vi "Mouse Monitor Terminate.vi"   [LabVIEW 2018]
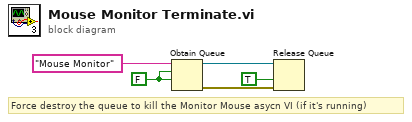
[diagram p0: block diagram]
diagram:
  w4 = FALSE ("create if not found? (T)")
  # "Force destroy the queue to kill the Monitor Mouse asycn VI (if it's running)"
  n1 = Obtain Queue(name (unnamed)="Mouse Monitor", element data type=w4, create if not found? (T)=w4) -> (queue out=w3:refnum<queue>, error out=w2:errorcluster)  [unwired: 2 in, 1 out]
  n2 = Release Queue(queue=w3, force destroy? (F)=TRUE, error in (no error)=w2) -> ()  [unwired: 3 out]
